vi "Set Calling VI Wnd Top and Active.vi"(8 "Error In":errorcluster) -> (0 "Error Out":errorcluster)   [LabVIEW 2016]
doc: "Sets the Caller VIs front panel Top (other windows can be moved in front), Active (title bar is selected), and gives Focus (keystrokes are directed to the panel).\n\nCopyright © 2010 Blue Ridge Test, Inc.\nwww.BlueRidgeTest.com"
uses:
  user32.dll
panel:
  out "Show\\Rest":i32
  out "Minimized?":i32
  out "FG hWnd":i32
  out "FG ProcID":i32
  out "hWnd ProcID":i32
  out "SetFG\\Attach":i32
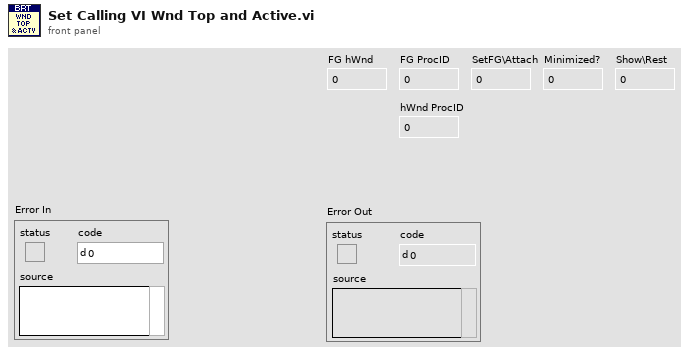
[diagram p1: front panel]
types:
  T1 = enum32{"Invalid", "Standard", "Closed", "Hidden", "Minimized", "Maximized"}
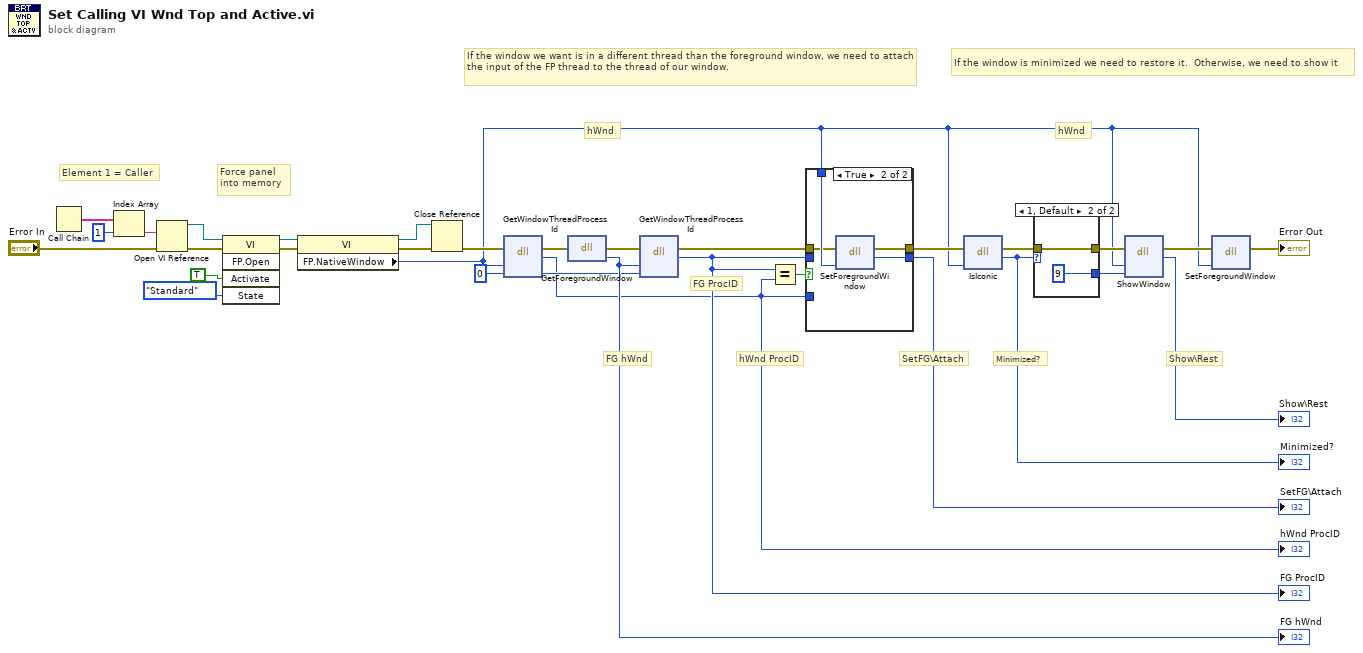
[diagram p0: block diagram]
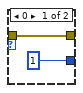
[diagram p2: hidden frame]
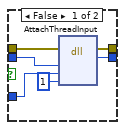
[diagram p3: hidden frame]
diagram:
  w20 = 0 ("lpdwProcessID")
  # "hWnd ProcID"
  # "Show\\Rest"
  # "Minimized?"
  # "SetFG\\Attach"
  # "Force panel\ninto memory"
  # "FG hWnd"
  # "FG ProcID"
  # "hWnd"
  # "If the window is minimized we need to restore it.  Otherwise, we need to show it"
  # "hWnd"
  # "If the window we want is in a different thread than the foreground window, we need to attach the input of the FP thread to the thread of our window."
  # "Element 1 = Caller"
  n1 = Call Chain() -> (call chain=w28:string[])
  n2 = Index Array(array=w28, index=1) -> (element=w27:string)
  n3 = Open VI Reference(vi path=w27, error in (no error)="Error In") -> (vi reference=w24:refnum<vi>, error out=w25:errorcluster)  [unwired: 4 in]
  n4 = invoke class="VI" method="FP.Open"(reference=w24, error in=w25, "Activate"=TRUE ("Activate?"), "State"=T1."Standard") -> (reference out=w5:refnum<vi>, error out=w6:errorcluster)  [unwired: 1 in, 3 out]
  n5 = property class="VI"(reference=w5, error in=w6) -> (reference out=w3:refnum<vi>, error out=w4:errorcluster, "FP.NativeWindow"=w1:u64)
  n6 = Close Reference(reference=w3, error in (no error)=w4) -> (error out=w2:errorcluster)
  n7 = dll-call lib="user32" fn="GetWindowThreadProcessId" label="Get\nWindow\nThread\nProcess\nId"(error in=w2, "hWnd"=w1, "lpdwProcessID"=w20) -> (error out=w15:errorcluster, w14:i32)  [unwired: 4 in, 1 out]
  "hWnd ProcID" <- w14
  n8 = dll-call lib="user32" fn="GetForegroundWindow" label="Get\nForeground\nWindow"(error in=w15) -> (error out=w16:errorcluster, "hWnd"=w21:i32)  [unwired: 2 in, 1 out]
  "FG hWnd" <- w21
  n9 = dll-call lib="user32" fn="GetWindowThreadProcessId" label="Get\nWindow\nThread\nProcess\nId"(error in=w16, "hWnd"=w21, "lpdwProcessID"=w20) -> (error out=w13:errorcluster, w18:i32)  [unwired: 4 in, 1 out]
  "FG ProcID" <- w18
  n10 = Equal?(x=w18, y=w14) -> (x = y?=w19:bool)
  n11 = case shown="True" w19 {
    tunnel: w18 -> [w37 _]
    tunnel: w14 -> [w36 _]
    tunnel: w1 -> [_ w41]
    tunnel: [w34 w40] -> w17
    tunnel: w13 -> [w33 w39]
    tunnel: [w32 w38] -> w23
    frame False {
      n12 = dll-call lib="user32" fn="AttachThreadInput" label="Attach\nThread\nInput"(error in=w33, "idAttach"=w37, "idAttachTo"=w36, "fAttach"=1) -> (error out=w32:errorcluster, w34:i32)  [unwired: 5 in, 1 out]
    }
    frame True {
      n13 = dll-call lib="user32" fn="SetForegroundWindow" label="Set\nForeground\nWindow"(error in=w39, "hWnd"=w41) -> (error out=w38:errorcluster, w40:i32)  [unwired: 3 in, 1 out]
    }
  }
  "SetFG\\Attach" <- w17
  n14 = dll-call lib="user32" fn="IsIconic"(error in=w23, "hWnd"=w1) -> (error out=w8:errorcluster, w12:i32)  [unwired: 3 in, 1 out]
  "Minimized?" <- w12
  n15 = case shown="1, Default" w12 {
    tunnel: [i16 1 ("nCmdshow") i16 9 ("nCmdshow")] -> w11
    tunnel: [w42 w44] -> w9
    tunnel: w8 -> [w42 w44]
    frame 0 {
    }
    frame 1, Default {
    }
  }
  n16 = dll-call lib="user32.dll" fn="ShowWindow"(error in=w9, "hWnd"=w1, "nCmdshow"=w11) -> (error out=w22:errorcluster, →"Show\\Rest":i32)  [unwired: 4 in, 1 out]
  n17 = dll-call lib="user32" fn="SetForegroundWindow" label="Set\nForeground\nWindow"(error in=w22, "hWnd"=w1) -> (error out=→"Error Out":errorcluster)  [unwired: 4 in, 1 out]
